vi "StackerStateMachine.vi"(0 "HMI to Control":T7, 1 "Arm Arrived":bool, 2 "StackClampState":T1, 5 "SensorInputData":T6, 7 "Intake Wheel State":T3, 9 "Tusk State":T4, 11 "error in":errorcluster) -> (4 "HMI to Control  Out":T7={"RightDriveValue"=0.0, "LeftDriveValue"=0.0, "Arm Manual "=0.0, "Stacker Manual "=0.0, "Claw Manual "=0.0, "ClawSlightOpenNumber"=0, "Intake Value "=0.0, "Arm States"=enum."4 Tote", "Claw States"=enum."Claw Manual ", "Intake Man. or Sense"=enum."Sensing", "Stacker in Manual?"=FALSE, "Drop Stack? "=FALSE, "Tusk Up Request"=FALSE, "Tusk Down Request"=FALSE, "Inver. Wheels  In Request"=FALSE, "Inverse. Wheels Out Request "=FALSE, "Get Out of Manual Control"=FALSE, "Exit Score State"=FALSE, "DriveStraight Help?"=FALSE, "Stacker Shut Off No."=0, "Stacker Need Off?"=FALSE, "Collecting?"=FALSE, "Go to Hover"=FALSE, "Stack Clamp Lock "=FALSE, "Stack Clamp Unlock "=FALSE, "Claw Intake Value "=0.0, "Stack Clamp Lock No. "=0}, 6 "SensorInputData out":T6, 8 "# of Totes Out":i32, 10 "Stacker State to Index":T5=enum."Hold", 12 "Tusk State to Actuate":T4, 13 "StackClampState to Actuate":T1, 14 "Intake Wheel State to Actuate":T3, 15 "error out":errorcluster)   [LabVIEW 2014]
uses:
  Typedefs/StackerStates.ctl
  Typedefs/HMI_to_Control.ctl
  Typedefs/Arm States.ctl
  Typedefs/ClawStates.ctl
  Typedefs/IntakeWheelSenseOrManual.ctl
  Typedefs/SensorInputData.ctl
  Typedefs/TuskStates.ctl
  Typedefs/IntakeWheelStates.ctl
  Typedefs/StackClampStates.ctl
  Typedefs/ClawStateMachine.ctl
  Gensubs/Bert_or_Ernie.vi
panel:
  in  "Ernie Needed Ranges":T2={"5 on ground upper range"=196.0, "5 on ground lower range"=182.0, "6 on ground upper range"=220.0, "6 on ground on lower range"=200.0, "Hold 4 Up Limit"=17.2, "Hold 4 Low Limit "=10.0, "Hold 5 Up Limit"=15.7, "Hold 5 Low Limit"=10.0, "Get Tote Upper Ok Range "=0.6, "Get Tote Lower Ok Range"=-2.0, "Drop Stack Upper Ok Range"=0.3, "Drop Stack Lower Ok Range"=-0.5, "6 Tote Cal Upper Range"=90.0, "6 Tote Cal Lower Range"=85.0, "5 Tote Cal Upper Range "=90.0, "5 Tote Cal Lower Range "=76.0, "Stacker on Ground Bottom #"=1.5, "Hold 4 on Ground Upper Range  "=172.0, "4 on ground U.R"=174.0, "4 on ground L.R"=165.0} {"4 on ground L.R" format="%#_13g"; "4 on ground U.R" format="%#_13g"; "6 Tote Cal Upper Range" format="%#_13g"}
  in  "Bert Needed Ranges":T2={"5 on ground upper range"=193.0, "5 on ground lower range"=176.0, "6 on ground upper range"=212.0, "6 on ground on lower range"=204.0, "Hold 4 Up Limit"=21.0, "Hold 4 Low Limit "=10.0, "Hold 5 Up Limit"=18.5, "Hold 5 Low Limit"=10.5, "Get Tote Upper Ok Range "=0.7, "Get Tote Lower Ok Range"=-2.0, "Drop Stack Upper Ok Range"=0.5, "Drop Stack Lower Ok Range"=-0.5, "6 Tote Cal Upper Range"=90.0, "6 Tote Cal Lower Range"=85.0, "5 Tote Cal Upper Range "=90.0, "5 Tote Cal Lower Range "=54.0, "Stacker on Ground Bottom #"=1.5, "Hold 4 on Ground Upper Range  "=172.0, "4 on ground U.R"=174.0, "4 on ground L.R"=157.0} {"4 on ground L.R" format="%#_13g"; "4 on ground U.R" format="%#_13g"; "6 Tote Cal Upper Range" format="%#_13g"}
  out "Stacker State Out":T5=enum."Hold"
  out "Stacker State In":T5
  # "When to \nadvance\nto \nother ranges\n\nHas to match\nsetpoints\nin stacker\nsub vi"
  # "4 Bar checks\nmust be \nin line with\ncals\nin 4 bar\nsub vi"
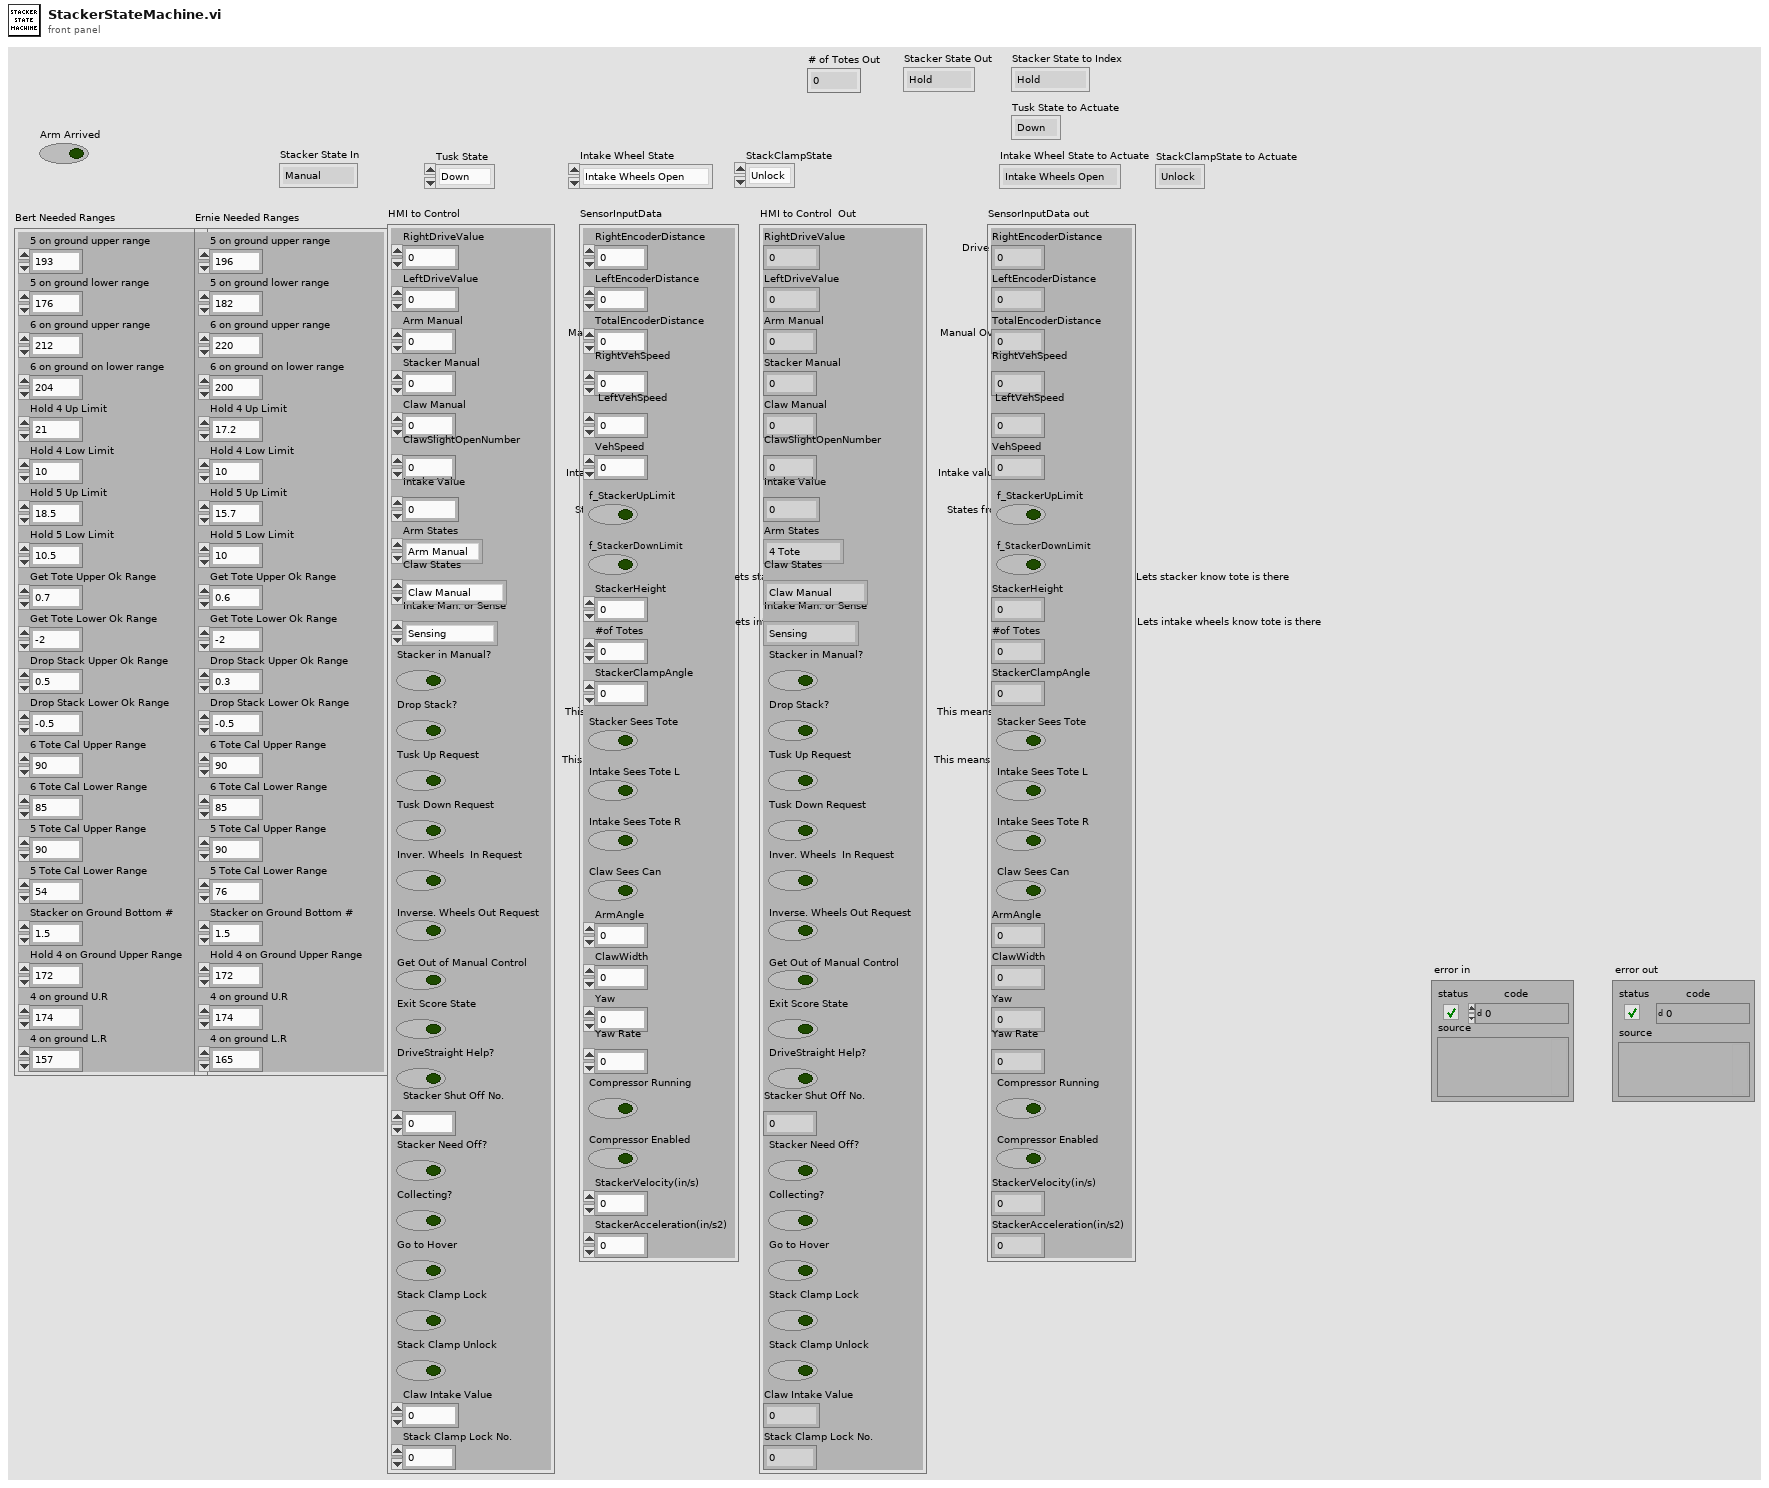
[diagram p1: front panel]
types:
  T1 = typedef "StackClampStates.ctl" = enum16{"Unlock", "Lock"}
  T2 = cluster{"5 on ground upper range":dbl, "5 on ground lower range":dbl, "6 on ground upper range":dbl, "6 on ground on lower range":dbl, "Hold 4 Up Limit":dbl, "Hold 4 Low Limit ":dbl, "Hold 5 Up Limit":dbl, "Hold 5 Low Limit":dbl, "Get Tote Upper Ok Range ":dbl, "Get Tote Lower Ok Range":dbl, "Drop Stack Upper Ok Range":dbl, "Drop Stack Lower Ok Range":dbl, "6 Tote Cal Upper Range":dbl, "6 Tote Cal Lower Range":dbl, "5 Tote Cal Upper Range ":dbl, "5 Tote Cal Lower Range ":dbl, "Stacker on Ground Bottom #":dbl, "Hold 4 on Ground Upper Range  ":dbl, "4 on ground U.R":dbl, "4 on ground L.R":dbl}
  T3 = typedef "IntakeWheelStates.ctl" = enum16{"Intake Wheels Open", "Intake Wheels Closed", "Decide off of Input", "Delay before Close", "Operator Request"}
  T4 = typedef "TuskStates.ctl" = enum16{"Down", "Up"}
  T5 = typedef "StackerStates.ctl" = enum16{"Manual ", "Hold", "Hold5", "Hold6", "GetTote", "DropStack", "Hover", "Hover5", "Wait for Up", "DecideHold", "DownTimerPeriod", "Prep Intake for Drop", "Check Arm before 5", "Make Arm ready for 5", "Check Arm before 6", "Make Arm ready for 6", "Delay for 5", "Delay for 6"}
  T6 = typedef "SensorInputData.ctl" = cluster{"RightEncoderDistance":dbl, "LeftEncoderDistance":dbl, "TotalEncoderDistance":dbl, "RightVehSpeed":dbl, "LeftVehSpeed":dbl, "VehSpeed":dbl, "f_StackerUpLimit":bool, "f_StackerDownLimit":bool, "StackerHeight":dbl, "#of Totes":u8, "StackerClampAngle":dbl, "Stacker Sees Tote":bool, "Intake Sees Tote L":bool, "Intake Sees Tote R":bool, "Claw Sees Can":bool, "ArmAngle":dbl, "ClawWidth":dbl, "Yaw":dbl, "Yaw Rate":dbl, "Compressor Running":bool, "Compressor Enabled":bool, "StackerVelocity(in/s)":dbl, "StackerAcceleration(in/s2)":dbl}
  T7 = typedef "HMI_to_Control.ctl" = cluster{"RightDriveValue":dbl, "LeftDriveValue":dbl, "Arm Manual ":dbl, "Stacker Manual ":dbl, "Claw Manual ":dbl, "ClawSlightOpenNumber":i8, "Intake Value ":sgl, "Arm States":T8, "Claw States":T9, "Intake Man. or Sense":T10, "Stacker in Manual?":bool, "Drop Stack? ":bool, "Tusk Up Request":bool, "Tusk Down Request":bool, "Inver. Wheels  In Request":bool, "Inverse. Wheels Out Request ":bool, "Get Out of Manual Control":bool, "Exit Score State":bool, "DriveStraight Help?":bool, "Stacker Shut Off No.":i8, "Stacker Need Off?":bool, "Collecting?":bool, "Go to Hover":bool, "Stack Clamp Lock ":bool, "Stack Clamp Unlock ":bool, "Claw Intake Value ":sgl, "Stack Clamp Lock No. ":i8}
  T8 = typedef "Arm States.ctl" = enum16{"Arm Manual ", "Ground", "Step", "1 Tote", "2 Tote", "3 Tote", "4 Tote", "5 Tote", "6 Tote", "Flip Can Arm", "Grab Can in auto", "Nudge"}
  T9 = typedef "ClawStates.ctl" = enum16{"Claw Manual ", "Claw Open", "Claw Closed", "Claw Slight Open", "Flip Can"}
  T10 = typedef "IntakeWheelSenseOrManual.ctl" = enum16{"Sensing", "Manual "}
  T11 = typedef "ClawStateMachine.ctl" = enum16{"Claw User Control", "Claw State Closed", "Claw State Slight Open"}
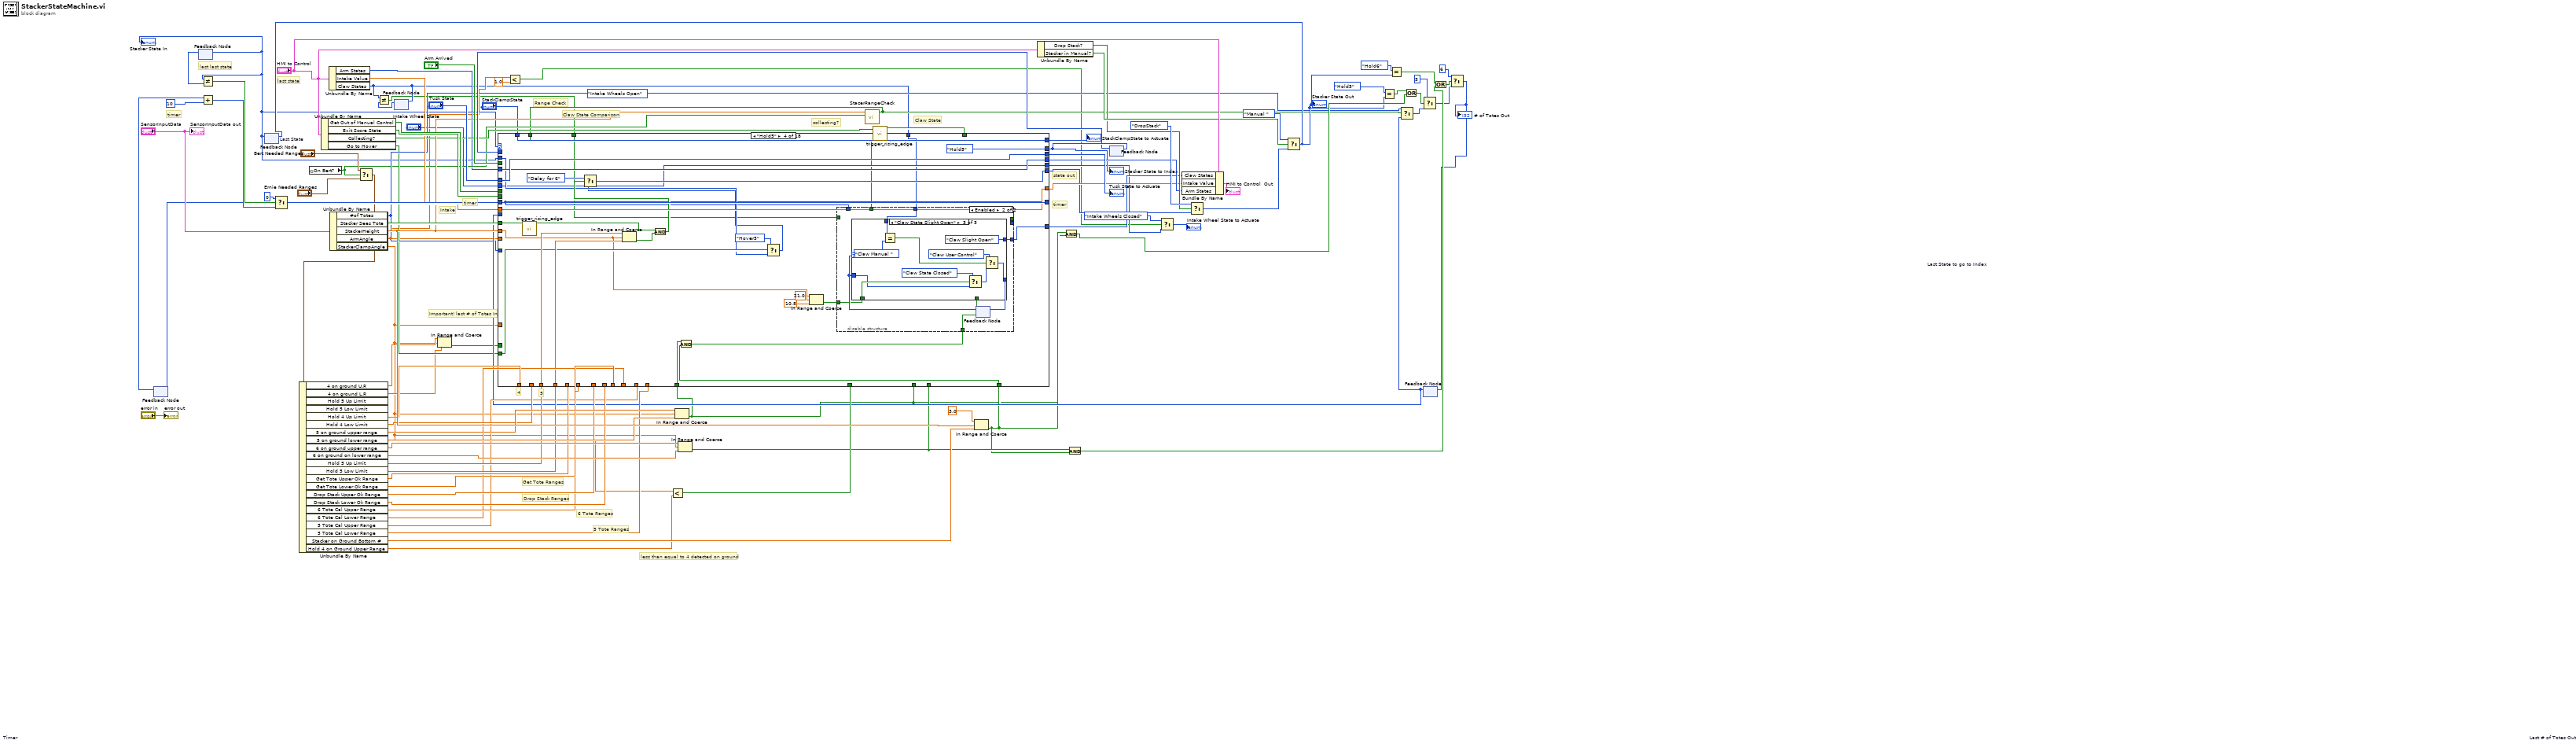
[diagram p0: block diagram]
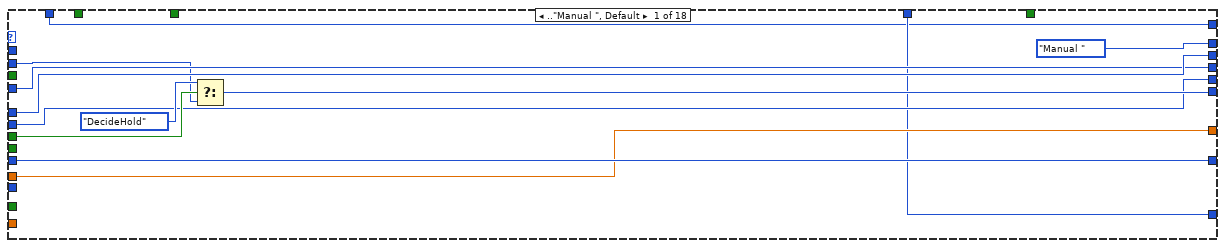
[diagram p2: hidden frame]
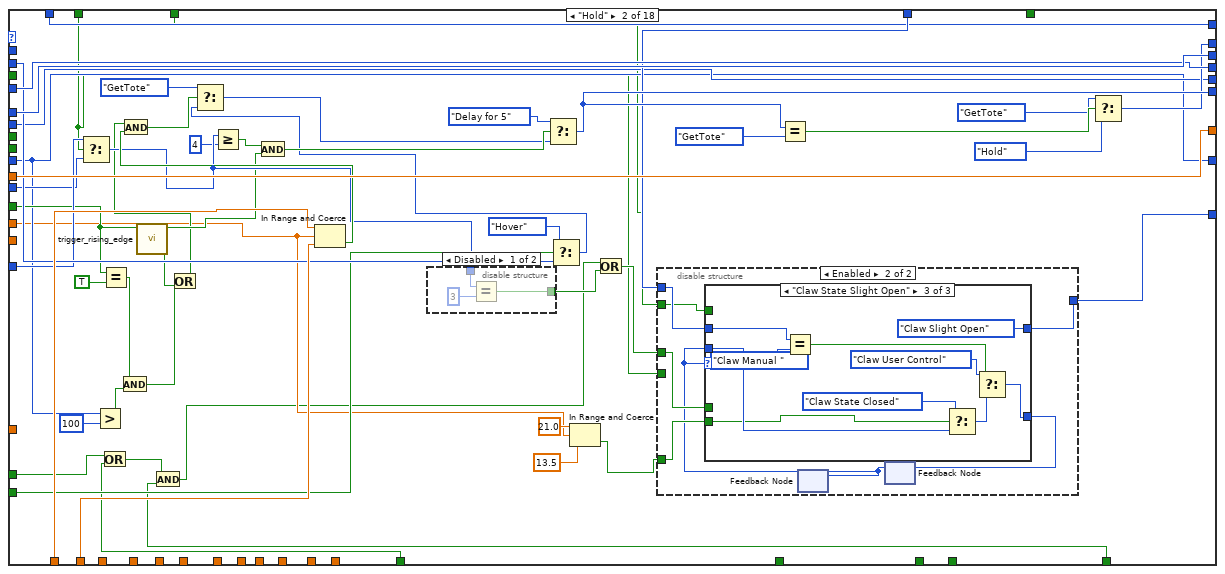
[diagram p3: hidden frame]
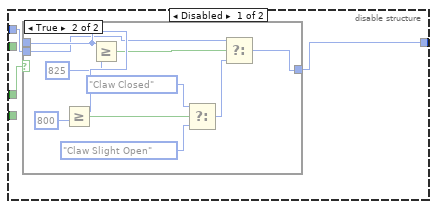
[diagram p4: hidden frame]
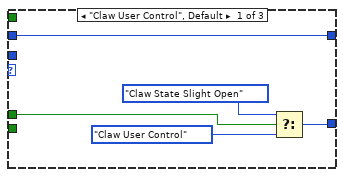
[diagram p6: hidden frame]
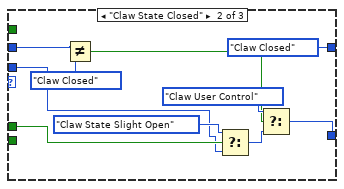
[diagram p7: hidden frame]
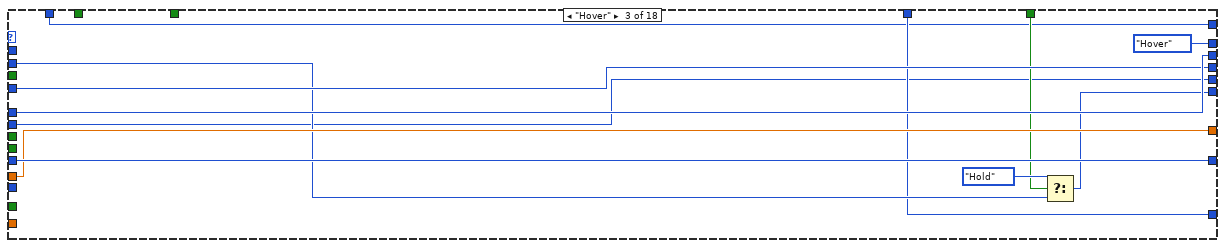
[diagram p9: hidden frame]
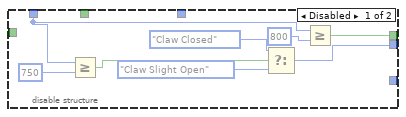
[diagram p10: hidden frame]
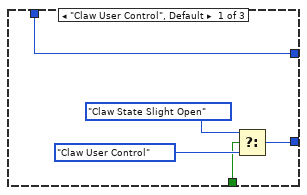
[diagram p11: hidden frame]
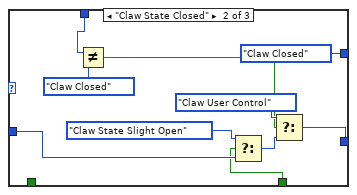
[diagram p12: hidden frame]
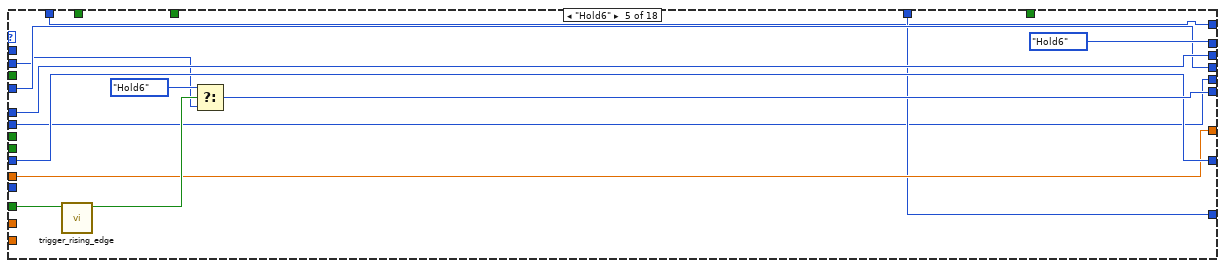
[diagram p13: hidden frame]
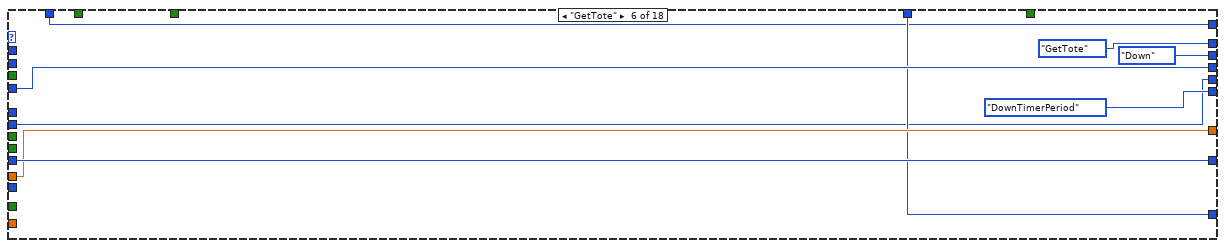
[diagram p14: hidden frame]
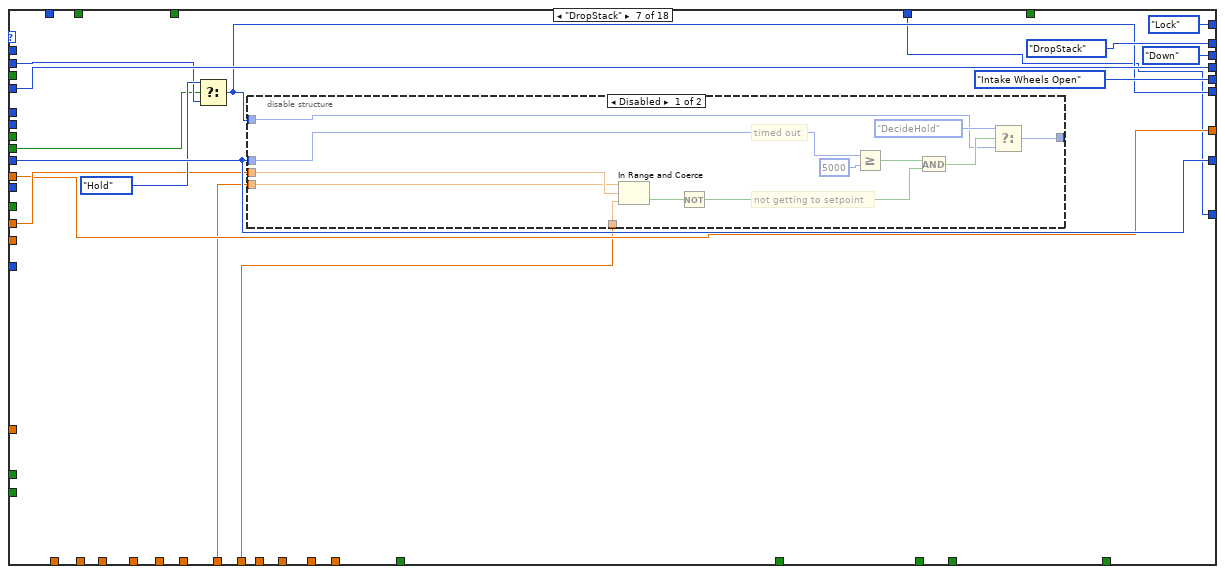
[diagram p15: hidden frame]
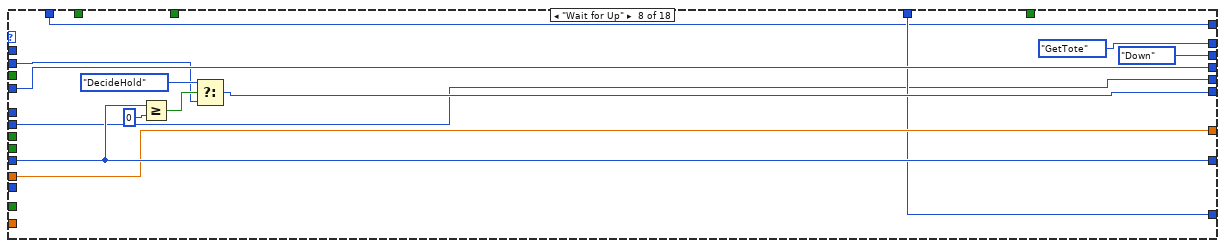
[diagram p17: hidden frame]
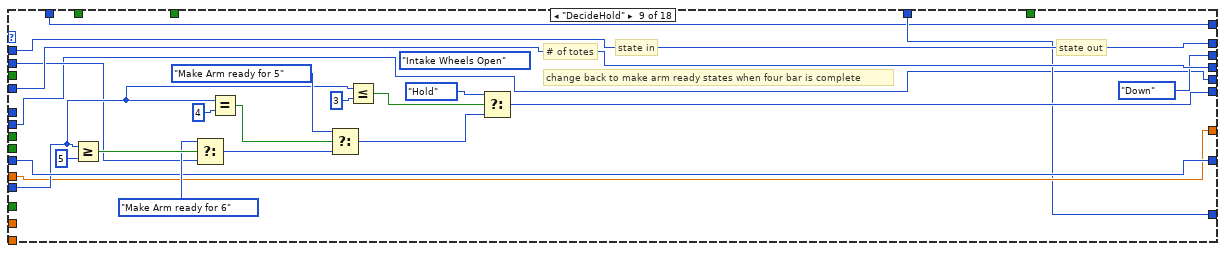
[diagram p18: hidden frame]
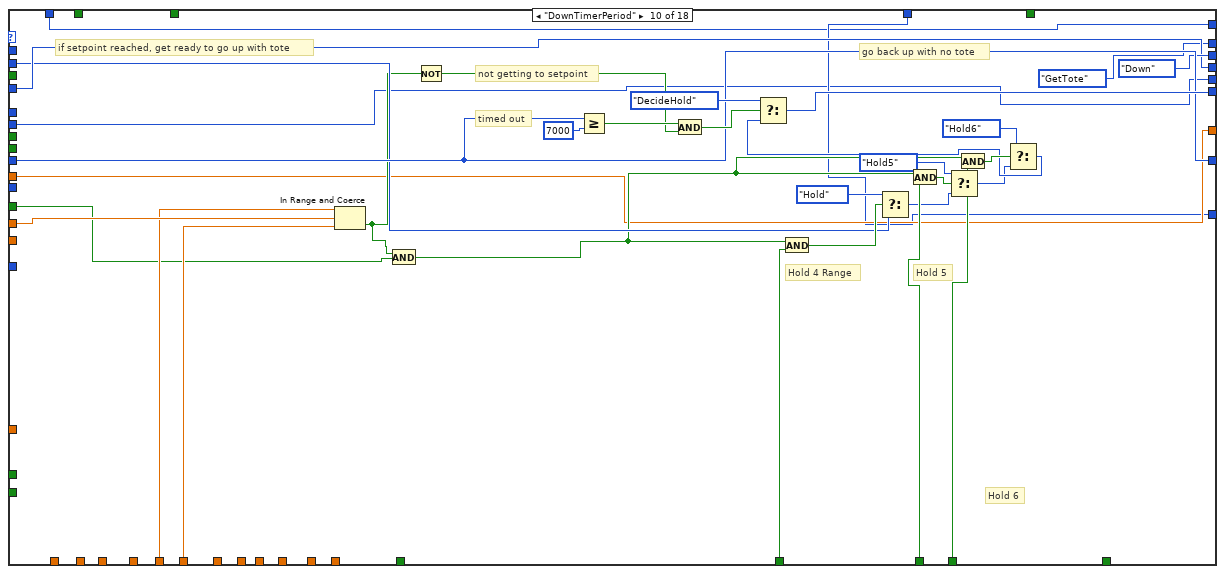
[diagram p19: hidden frame]
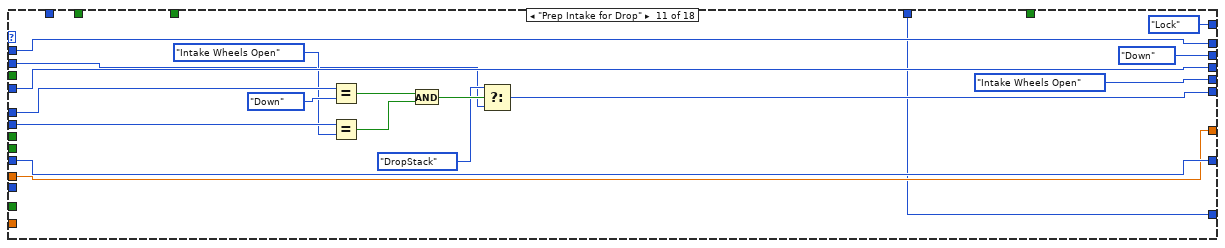
[diagram p20: hidden frame]
diagram:
  (unwired) IntakeWheelStates."Intake Wheels Open" ("y")
  # "Claw State Comparison"
  # "Range Check"
  # "Claw State"
  # "collecting?"
  # "less than equal to 4 detected on ground"
  # "5 Tote Ranges"
  # "6 Tote Ranges"
  # "Drop Stack Ranges"
  # "Get Tote Ranges"
  # "5"
  # "4"
  # "timer"
  # "state out"
  # "Important! last # of Totes In"
  # "Intake"
  # "timer"
  # "last state"
  # "last last state"
  # "timer"
  n1 = feedback #1 "Timer"() -> (w75:u32)  [unwired: 1 in]
  n2 = feedback #2() -> (w73:T5)  [unwired: 1 in]
  n3 = Add(x=w75, y=u32 10) -> (x+y=w91:u32)
  n4 = feedback #3 "Last State"() -> (w19:T5)  [unwired: 1 in]
  "Stacker State In" <- w19
  n5 = feedback-in #2(w19) -> ()
  n6 = Not Equal?(x=w19, y=w73) -> (x != y?=w90:bool)
  n7 = Select(t=u32 0, s=w90, f=w91) -> (s? t:f=w72:u32)
  n8 = global read "Bert_or_Ernie.vi" "On Bert?"() -> (w25:bool)
  n9 = Unbundle By Name("HMI to Control") -> ("Get Out of Manual Control"=w79:bool, "Exit Score State"=w78:bool, "Collecting?"=w29:bool, "Go to Hover"=w26:bool)
  n10 = Unbundle By Name("HMI to Control") -> ("Arm States"=w16:T8, "Intake Value"=w69:sgl, "Claw States"=w9:T9)
  n11 = Unbundle By Name("SensorInputData") -> ("#of Totes"=w27:u8, "Stacker Sees Tote"=w71:bool, "StackerHeight"=w67:dbl, "ArmAngle"=w12:dbl, "StackerClampAngle"=w2:dbl)
  n12 = Select(t="Bert Needed Ranges", s=w25, f="Ernie Needed Ranges") -> (s? t:f=w48:T2)
  n13 = Unbundle By Name(w48) -> ("4 on ground U.R"=w4:dbl, "4 on ground L.R"=w3:dbl, "Hold 4 Up Limit"=w61:dbl, "Hold 4 Low Limit"=w60:dbl, "5 on ground upper range"=w66:dbl, "5 on ground lower range"=w64:dbl, "6 on ground upper range"=w63:dbl, "6 on ground on lower range"=w62:dbl, "Hold 5 Up Limit"=w59:dbl, "Hold 5 Low Limit"=w58:dbl, "Get Tote Upper Ok Range"=w57:dbl, "Get Tote Lower Ok Range"=w56:dbl, "Drop Stack Upper Ok Range"=w55:dbl, "Drop Stack Lower Ok Range"=w54:dbl, "6 Tote Cal Upper Range"=w53:dbl, "6 Tote Cal Lower Range"=w52:dbl, "5 Tote Cal Upper Range"=w51:dbl, "5 Tote Cal Lower Range"=w50:dbl, "Stacker on Ground Bottom #"=w33:dbl, "Hold 4 on Ground Upper Range"=w32:dbl)  [unwired: 2 out]
  n14 = feedback-in #4(w9) -> ()
  n15 = feedback #4() -> (w8:T9)  [unwired: 1 in]
  n16 = Not Equal?(x=w9, y=w8) -> (x != y?=w7:bool)
  n17 = In Range and Coerce(upper limit=w4, x=w2, lower limit=w3) -> (In Range?=w6:bool)  [unwired: 1 out]
  n18 = Less?(x=w12, y=1.0) -> (x < y?=w10:bool)
  n19 = Less?(x=w2, y=w32) -> (x < y?=w31:bool)
  n20 = In Range and Coerce(upper limit=w66, x=w2, lower limit=w64) -> (In Range?=w1:bool)  [unwired: 1 out]
  n21 = In Range and Coerce(upper limit=w63, x=w2, lower limit=w62) -> (In Range?=w24:bool)  [unwired: 1 out]
  n22 = call "StacerRangeCheck.vi"("On Bert?"=w25, "Stacker"=w67) -> ("In ok range to count?"=w23:bool)  [unwired: 9 in]
  n23 = call "trigger_rising_edge.vi"("input"=w29) -> ("rising"=w21:bool)  [unwired: 10 in]
  n24 = In Range and Coerce(upper limit=3.0, x=w67, lower limit=w33) -> (In Range?=w5:bool)  [unwired: 1 out]
  n25 = Unbundle By Name("HMI to Control") -> ("Drop Stack?"=w84:bool, "Stacker in Manual?"=w88:bool)
  n26 = And(x=w5, y=w1) -> (x .and. y?=w45:bool)
  n27 = And(x=w24, y=w5) -> (x .and. y?=w36:bool)
  n28 = feedback #5 "Last State to go to Index"() -> (w74:T5)  [unwired: 1 in]
  n29 = feedback #6 "Last # of Totes Out"() -> (w28:i32)  [unwired: 1 in]
  n30 = case shown="\"Hold5\"" w19 {
    tunnel: [w105 w149 w213 w250 w302 StackerStates."DownTimerPeriod" ("Enum") w321 w349 w364 w403 w414 w431 w450 w472 w486 w512 w530 w554] -> w30
    tunnel: w71 -> [_ w129 _ w249 w299 _ _ _ _ w389 _ _ _ _ _ _ _ _]
    tunnel: w72 -> [w104 w126 w221 w235 w301 w312 w324 w348 w363 w401 w412 w430 w455 w470 w496 w511 w531 w545]
    tunnel: [w104 w126 w221 w235 w301 w312 w324 w348 w363 w401 w412 w430 w455 w470 w496 w511 w531 w545] -> w77
    tunnel: [StackerStates."Manual " ("State In 2") w145 StackerStates."Hover" ("t") StackerStates."Hold5" ("Enum") StackerStates."Hold6" ("Enum") StackerStates."GetTote" ("State In 2") StackerStates."DropStack" ("State In 2") StackerStates."GetTote" ("State In 2") w362 StackerStates."GetTote" ("State In 2") w413 StackerStates."GetTote" ("State In 2") w445 StackerStates."GetTote" ("State In 2") w481 w519 w527 StackerStates."Hover" ("t")] -> w76
    tunnel: "Tusk State" -> [w103 w159 w219 w251 w300 _ _ _ _ _ w422 _ _ _ _ w518 w526 w551]
    tunnel: "Intake Wheel State" -> [w102 w131 w210 w233 w291 w304 _ w340 w353 w375 w420 _ _ _ _ w516 w524 w538]
    tunnel: [w103 w159 w219 w251 w300 TuskStates."Down" ("Tusk State") TuskStates."Down" ("Tusk State") TuskStates."Down" ("Tusk State") TuskStates."Down" ("Tusk State") TuskStates."Down" ("Tusk State") TuskStates."Down" ("Tusk State") TuskStates."Down" ("Tusk State") TuskStates."Down" ("Tusk State") TuskStates."Down" ("Tusk State") TuskStates."Down" ("Tusk State") w518 w526 w551] -> w82
    tunnel: [w102 w131 w210 w233 w291 w304 IntakeWheelStates."Intake Wheels Open" ("Intake Wheel States") w340 w353 w375 IntakeWheelStates."Intake Wheels Open" ("Intake Wheel States") IntakeWheelStates."Intake Wheels Closed" ("Intake Wheel States") IntakeWheelStates."Intake Wheels Closed" ("Intake Wheel States") IntakeWheelStates."Intake Wheels Closed" ("Intake Wheel States") IntakeWheelStates."Intake Wheels Closed" ("Intake Wheel States") w516 w524 w538] -> w14
    tunnel: w74 -> [_ _ _ _ _ _ _ _ w362 _ w413 _ w446 _ w482 w519 w527 _]
    tunnel: w16 -> [w101 w158 w218 w246 w295 w308 w326 w345 w361 w399 w425 w433 w460 w473 w493 w517 w525 w552]
    tunnel: [w101 w158 w218 w246 w295 w308 w326 w345 w361 w399 w425 w429 w458 w469 w497 w517 w525 w552] -> w81
    tunnel: "Arm Arrived" -> [_ _ _ _ _ _ _ _ _ _ _ _ _ _ _ _ _ _]
    tunnel: w79 -> [w107 _ _ _ _ _ _ _ _ _ _ _ _ _ _ _ _ _]
    tunnel: w67 -> [_ w118 _ w224 _ _ w322 _ _ w398 _ _ _ _ _ w507 w528 _]
    tunnel: w78 -> [_ _ _ _ _ _ w314 _ _ _ _ _ _ _ _ _ _ _]
    tunnel: w28 -> [_ w136 _ _ _ _ _ _ w359 _ _ _ _ _ _ _ _ _]
    tunnel: [w100 w157 w217 w248 w297 w307 w320 w343 w356 w381 w411 w428 w454 w466 w492 w515 w529 w553] -> w70
    tunnel: w69 -> [w100 w157 w217 w248 w297 w307 w320 w343 w356 w381 w411 w428 w454 w466 w492 w515 w529 w553]
    tunnel: w12 -> [_ _ _ _ _ _ _ _ _ _ _ _ w453 _ w491 _ _ _]
    tunnel: w19 -> [w99 w142 w215 w237 w294 _ w319 w344 w357 w392 w410 _ w451 _ w489 w506 w532 w555]
    tunnel: w61 -> [_ w151 _ _ _ _ _ _ _ _ _ _ _ _ _ w505 _ _]
    tunnel: w60 -> [_ w150 _ _ _ _ _ _ _ _ _ _ _ _ _ w504 _ _]
    tunnel: w59 -> [_ _ _ w244 _ _ _ _ _ _ _ _ _ _ _ _ w523 _]
    tunnel: w58 -> [_ _ _ w243 _ _ _ _ _ _ _ _ _ _ _ _ w522 _]
    tunnel: w57 -> [_ _ _ _ _ _ _ _ _ w396 _ _ _ _ _ _ _ _]
    tunnel: w56 -> [_ _ _ _ _ _ _ _ _ w395 _ _ _ _ _ _ _ _]
    tunnel: w55 -> [_ _ _ _ _ _ w318 _ _ _ _ _ _ _ _ _ _ _]
    tunnel: w54 -> [_ _ _ _ _ _ w317 _ _ _ _ _ _ _ _ _ _ _]
    tunnel: w53 -> [_ _ _ _ _ _ _ _ _ _ _ _ w444 _ w488 _ _ _]
    tunnel: w52 -> [_ _ _ _ _ _ _ _ _ _ _ _ w443 _ w487 _ _ _]
    tunnel: w51 -> [_ _ _ _ _ _ _ _ _ _ _ _ _ _ _ _ _ _]
    tunnel: w50 -> [_ _ _ _ _ _ _ _ _ _ _ _ _ _ _ _ _ _]
    tunnel: w31 -> [_ _ _ _ _ _ _ _ _ w394 _ _ _ _ _ _ _ _]
    tunnel: w1 -> [_ _ _ _ _ _ _ _ _ w383 _ _ _ _ _ _ _ _]
    tunnel: w24 -> [_ _ _ _ _ _ _ _ _ w384 _ _ _ _ _ _ _ _]
    tunnel: w21 -> [_ _ w214 _ _ _ _ _ _ _ _ _ _ _ _ _ _ w556]
    tunnel: w27 -> [_ w137 _ _ _ _ _ _ _ _ _ _ _ _ _ _ _ _]
    tunnel: w26 -> [_ w140 _ w238 _ _ _ _ _ _ _ _ _ _ _ _ _ _]
    tunnel: [w98 w138 w212 w222 w293 w306 w315 w342 w355 w377 w409 w427 w442 w465 w480 w503 w521 w540] -> w20
    tunnel: w9 -> [w98 w139 w212 w230 w293 w306 w315 w342 w355 w377 w409 w427 w442 w465 w480 w503 w521 w541]
    tunnel: w23 -> [_ w121 _ w232 _ _ _ _ _ _ _ _ _ _ _ _ _ _]
    tunnel: "StackClampState" -> [w97 w132 w211 w234 w292 w305 _ w341 w354 w376 _ w426 w441 w464 w479 w502 w520 w539]
    tunnel: [w97 w132 w211 w234 w292 w305 StackClampStates."Lock" ("StackClampState") w341 w354 w376 StackClampStates."Lock" ("StackClampState") w426 w441 w464 w479 w502 w520 w539] -> w17
    tunnel: w7 -> [_ w122 _ w231 _ _ _ _ _ _ _ _ _ _ _ _ _ _]
    tunnel: w6 -> [_ w112 _ _ _ _ _ _ _ _ _ _ _ _ _ _ _ _]
    tunnel: w5 -> [_ w117 _ w229 _ _ _ _ _ _ _ _ _ _ _ _ _ _]
    tunnel: w2 -> [_ _ _ _ _ _ _ _ _ _ _ _ _ _ _ _ _ _]
    tunnel: w1 -> [_ w110 _ w223 _ _ _ _ _ _ _ _ _ _ _ _ _ _]
    frame .."Manual ", Default {
      n31 = Select(t=StackerStates."DecideHold" ("State In 2"), s=w107, f=w99) -> (s? t:f=w105:T5)
    }
    frame "Hold" {
      n32 = Select(t=w137, s=w121, f=w136) -> (s? t:f=w135:i32)
      n33 = Greater?(x=w126, y=u32 100) -> (0:w113:bool)
      n34 = Or(x=w112, y=w110) -> (x .or. y?=w111:bool)
      n35 = Equal?(x=w129, y=TRUE) -> (x = y?=w127:bool)
      n36 = And(x=w127, y=w113) -> (x .and. y?=w124:bool)
      n37 = call "trigger_rising_edge.vi"("input"=w129) -> ("rising"=w130:bool)  [unwired: 10 in]
      n38 = And(x=w111, y=w117) -> (x .and. y?=w114:bool)
      n39 = Or(x=w124, y=w130) -> (x .or. y?=w123:bool)
      n40 = Greater Or Equal?(x=w135, y=u8 4) -> (x >= y?=w116:bool)
      n41 = And(x=w116, y=w130) -> (x .and. y?=w156:bool)
      n42 = In Range and Coerce(upper limit=w151, x=w118, lower limit=w150) -> (In Range?=w154:bool)  [unwired: 1 out]
      n43 = And(x=w123, y=w154) -> (x .and. y?=w153:bool)
      n44 = disable-structure shown="Disabled" {
        disable-tunnel: w135 -> [w209 _]
        disable-tunnel: [w208 _] -> w134
        frame Disabled {
          n45 = Equal?(x=w209, y=3) -> (x = y?=w208:bool)
        }
        frame Enabled {
        }
      }
      n46 = Select(t=StackerStates."Hover" ("y"), s=w140, f=w142) -> (s? t:f=w141:T5)
      n47 = Select(t=StackerStates."GetTote" ("State In 2"), s=w153, f=w141) -> (s? t:f=w155:T5)
      n48 = Select(t=StackerStates."Delay for 5" ("State In 2"), s=w156, f=w155) -> (s? t:f=w149:T5)
      n49 = In Range and Coerce(upper limit=21.0, x=w118, lower limit=13.5) -> (In Range?=w109:bool)  [unwired: 1 out]
      n50 = Or(x=w114, y=w134) -> (x .or. y?=w133:bool)
      n51 = disable-structure shown="Enabled" {
        disable-tunnel: w139 -> [w163 w181]
        disable-tunnel: [w162 w180] -> w138
        disable-tunnel: w133 -> [w161 w179]
        disable-tunnel: w122 -> [_ w176]
        disable-tunnel: w121 -> [_ _]
        disable-tunnel: w109 -> [_ w177]
        frame Disabled {
          n52 = case shown="True" w161 {
            tunnel: w163 -> [w164 w166]
            tunnel: _ -> [_ w170]
            tunnel: [w164 w165] -> w162
            frame False {
            }
            frame True {
              n53 = Greater Or Equal?(x=w170, y=u32 800) -> (x >= y?=w171:bool)
              n54 = Greater Or Equal?(x=w170, y=u32 825) -> (x >= y?=w168:bool)
              n55 = Select(t=ClawStates."Claw Closed" ("Claw States"), s=w171, f=ClawStates."Claw Slight Open" ("Claw States")) -> (s? t:f=w167:T9)
              n56 = Select(t=w166, s=w168, f=w167) -> (s? t:f=w165:T9)
            }
          }
        }
        frame Enabled {
          n57 = feedback #7() -> ()  [unwired: 2 in]
          n58 = feedback #8() -> (w175:T11)  [unwired: 1 in]
          n59 = case shown="\"Claw State Slight Open\"" w175 {
            tunnel: w181 -> [w186 w189 w202]
            tunnel: [w186 ClawStates."Claw Closed" ("Claw States") ClawStates."Claw Slight Open" ("Claw States")] -> w180
            tunnel: w179 -> [w184 w192 _]
            tunnel: [w182 w190 w197] -> w178
            tunnel: w177 -> [_ _ w203]
            tunnel: w175 -> [_ w191 w205]
            tunnel: w176 -> [_ _ _]
            frame "Claw User Control", Default {
              n60 = Select(t=ClawStateMachine."Claw State Slight Open", s=w184, f=ClawStateMachine."Claw User Control") -> (s? t:f=w182:T11)
            }
            frame "Claw State Closed" {
              n61 = Not Equal?(x=w189, y=ClawStates."Claw Closed") -> (x != y?=w187:bool)
              n62 = Select(t=ClawStateMachine."Claw State Slight Open", s=w192, f=w191) -> (s? t:f=w193:T11)
              n63 = Select(t=ClawStateMachine."Claw User Control", s=w187, f=w193) -> (s? t:f=w190:T11)
            }
            frame "Claw State Slight Open" {
              n64 = Equal?(x=w202, y=ClawStates."Claw Manual ") -> (x = y?=w198:bool)
              n65 = Select(t=ClawStateMachine."Claw State Closed", s=w203, f=w205) -> (s? t:f=w200:T11)
              n66 = Select(t=ClawStateMachine."Claw User Control", s=w198, f=w200) -> (s? t:f=w197:T11)
            }
          }
          n67 = feedback-in #7(w175) -> ()
          n68 = feedback-in #8(w178) -> ()
        }
      }
      n69 = Equal?(x=w149, y=StackerStates."GetTote") -> (x = y?=w147:bool)
      n70 = Select(t=StackerStates."GetTote" ("y"), s=w147, f=StackerStates."Hold" ("State In 2")) -> (s? t:f=w145:T5)
    }
    frame "Hover" {
      n71 = Select(t=StackerStates."Hold", s=w214, f=w215) -> (s? t:f=w213:T5)
    }
    frame "Hold5" {
      n72 = call "trigger_rising_edge.vi"("input"=w249) -> ("rising"=w241:bool)  [unwired: 10 in]
      n73 = In Range and Coerce(upper limit=w244, x=w224, lower limit=w243) -> (In Range?=w242:bool)  [unwired: 1 out]
      n74 = And(x=w241, y=w242) -> (x .and. y?=w240:bool)
      n75 = And(x=w223, y=w229) -> (x .and. y?=w228:bool)
      n76 = Select(t=StackerStates."Hover5" ("y"), s=w238, f=w237) -> (s? t:f=w236:T5)
      n77 = Select(t=StackerStates."Delay for 6" ("Enum"), s=w240, f=w236) -> (s? t:f=w250:T5)
      n78 = In Range and Coerce(upper limit=21.0, x=w224, lower limit=10.8) -> (In Range?=w225:bool)  [unwired: 1 out]
      n79 = disable-structure shown="Enabled" {
        disable-tunnel: w235 -> [w255 _]
        disable-tunnel: [w253 _] -> _
        disable-tunnel: [w252 _] -> _
        disable-tunnel: w232 -> [_ _]
        disable-tunnel: w231 -> [_ _]
        disable-tunnel: w230 -> [_ w265]
        disable-tunnel: w228 -> [_ w264]
        disable-tunnel: w225 -> [_ w261]
        disable-tunnel: [_ w260] -> w222
        frame Disabled {
          n80 = Greater Or Equal?(x=w255, y=u32 750) -> (x >= y?=w258:bool)
          n81 = Select(t=ClawStates."Claw Closed" ("Claw States"), s=w258, f=ClawStates."Claw Slight Open") -> (s? t:f=w252:T9)
          n82 = Greater Or Equal?(x=w255, y=u32 800) -> (x >= y?=w253:bool)
        }
        frame Enabled {
          n83 = feedback #9() -> (w262:T11)  [unwired: 1 in]
          n84 = case shown="\"Claw State Slight Open\"" w262 {
            tunnel: [w266 ClawStates."Claw Closed" ("Claw States") ClawStates."Claw Slight Open" ("Claw States")] -> w260
            tunnel: [w268 w276 w281] -> w263
            tunnel: w265 -> [w266 w273 w286]
            tunnel: w264 -> [w267 w271 _]
            tunnel: w262 -> [_ w272 w287]
            tunnel: w261 -> [_ _ w288]
            frame "Claw User Control", Default {
              n85 = Select(t=ClawStateMachine."Claw State Slight Open", s=w267, f=ClawStateMachine."Claw User Control") -> (s? t:f=w268:T11)
            }
            frame "Claw State Closed" {
              n86 = Not Equal?(x=w273, y=ClawStates."Claw Closed") -> (x != y?=w274:bool)
              n87 = Select(t=ClawStateMachine."Claw State Slight Open", s=w271, f=w272) -> (s? t:f=w277:T11)
              n88 = Select(t=ClawStateMachine."Claw User Control", s=w274, f=w277) -> (s? t:f=w276:T11)
            }
            frame "Claw State Slight Open" {
              n89 = Equal?(x=w286, y=ClawStates."Claw Manual ") -> (x = y?=w283:bool)
              n90 = Select(t=ClawStateMachine."Claw State Closed", s=w288, f=w287) -> (s? t:f=w282:T11)
              n91 = Select(t=ClawStateMachine."Claw User Control", s=w283, f=w282) -> (s? t:f=w281:T11)
            }
          }
          n92 = feedback-in #9(w263) -> ()
        }
      }
    }
    frame "Hold6" {
      n93 = call "trigger_rising_edge.vi"("input"=w299) -> ("rising"=w298:bool)  [unwired: 10 in]
      n94 = Select(t=StackerStates."Hold6" ("State Out 2"), s=w298, f=w294) -> (s? t:f=w302:T5)
    }
    frame "GetTote" {
    }
    frame "DropStack" {
      n95 = Select(t=StackerStates."Hold" ("Enum"), s=w314, f=w319) -> (s? t:f=w321:T5)
      n96 = disable-structure shown="Disabled" {
        disable-tunnel: [w333 _] -> _
        disable-tunnel: w324 -> [w332 _]
        disable-tunnel: w321 -> [w331 _]
        disable-tunnel: w322 -> [w330 _]
        disable-tunnel: w318 -> [w329 _]
        disable-tunnel: w317 -> [w328 _]
        frame Disabled {
          # "not getting to setpoint"
          # "timed out"
          n97 = In Range and Coerce(upper limit=w329, x=w330, lower limit=w328) -> (In Range?=w335:bool)  [unwired: 1 out]
          n98 = Not(x=w335) -> (.not. x?=w337:bool)
          n99 = Greater Or Equal?(x=w332, y=u32 5000) -> (x >= y?=w339:bool)
          n100 = And(x=w339, y=w337) -> (x .and. y?=w338:bool)
          n101 = Select(t=StackerStates."DecideHold" ("Stacker State In 2"), s=w338, f=w331) -> (s? t:f=w333:T5)
        }
        frame Enabled {
        }
      }
    }
    frame "Wait for Up" {
      n102 = Greater Or Equal?(x=w348, y=u32 0) -> (x >= y?=w351:bool)
      n103 = Select(t=StackerStates."DecideHold" ("Stacker State In 2"), s=w351, f=w344) -> (s? t:f=w349:T5)
    }
    frame "DecideHold" {
      (unwired) IntakeWheelStates."Intake Wheels Open" ("Intake Wheel States")
      # "# of totes"
      # "change back to make arm ready states when four bar is complete"
      # "state out"
      # "state in"
      n104 = Greater Or Equal?(x=w359, y=i8 5) -> (x >= y?=w374:bool)
      n105 = Select(t=StackerStates."Make Arm ready for 6" ("State In 2"), s=w374, f=w357) -> (s? t:f=w372:T5)
      n106 = Equal?(x=w359, y=i8 4) -> (x = y?=w370:bool)
      n107 = Select(t=StackerStates."Make Arm ready for 5" ("State In 2"), s=w370, f=w372) -> (s? t:f=w367:T5)
      n108 = Less Or Equal?(x=w359, y=i8 3) -> (x <= y?=w365:bool)
      n109 = Select(t=StackerStates."Hold" ("State In 2"), s=w365, f=w367) -> (s? t:f=w364:T5)
    }
    frame "DownTimerPeriod" {
      # "Hold 5"
      # "Hold 6"
      # "Hold 4 Range"
      # "if setpoint reached, get ready to go up with tote"
      # "go back up with no tote"
      # "not getting to setpoint"
      # "timed out"
      n110 = In Range and Coerce(upper limit=w396, x=w398, lower limit=w395) -> (In Range?=w390:bool)  [unwired: 1 out]
      n111 = And(x=w390, y=w389) -> (x .and. y?=w385:bool)
      n112 = Not(x=w390) -> (.not. x?=w405:bool)
      n113 = Greater Or Equal?(x=w401, y=u32 7000) -> (x >= y?=w407:bool)
      n114 = And(x=w407, y=w405) -> (x .and. y?=w406:bool)
      n115 = And(x=w385, y=w394) -> (x .and. y?=w393:bool)
      n116 = Select(t=StackerStates."Hold", s=w393, f=w392) -> (s? t:f=w379:T5)
      n117 = And(x=w385, y=w383) -> (x .and. y?=w388:bool)
      n118 = Select(t=StackerStates."Hold5", s=w388, f=w379) -> (s? t:f=w380:T5)
      n119 = And(x=w385, y=w384) -> (x .and. y?=w386:bool)
      n120 = Select(t=StackerStates."Hold6", s=w386, f=w380) -> (s? t:f=w382:T5)
      n121 = Select(t=StackerStates."DecideHold" ("Stacker State In 2"), s=w406, f=w382) -> (s? t:f=w403:T5)
    }
    frame "Prep Intake for Drop" {
      n122 = Equal?(x=w422, y=TuskStates."Down") -> (x = y?=w418:bool)
      n123 = Equal?(x=w420, y=IntakeWheelStates."Intake Wheels Open") -> (x = y?=w417:bool)
      n124 = And(x=w418, y=w417) -> (x .and. y?=w416:bool)
      n125 = Select(t=StackerStates."DropStack" ("Enum"), s=w416, f=w410) -> (s? t:f=w414:T5)
    }
    frame "Check Arm before 5" {
      # "Arm State"
      # "Stacker State"
      # "timer"
      # "state to index"
      n126 = Equal?(x=w433, y=Arm_States."6 Tote") -> (x = y?=w436:bool)
      n127 = Select(t=w433, s=w436, f=Arm_States."6 Tote") -> (s? t:f=w429:T8)
      n128 = Select(t=StackerStates."Hold5" ("Enum"), s=w436, f=StackerStates."Make Arm ready for 5") -> (s? t:f=w431:T5)
    }
    frame "Make Arm ready for 5" {
      # "Stacker State"
      # "Arm State"
      # "timer"
      n129 = Equal?(x=w460, y=Arm_States."6 Tote") -> (x = y?=w461:bool)
      n130 = Select(t=w460, s=w461, f=Arm_States."6 Tote") -> (s? t:f=w458:T8)
      n131 = In Range and Coerce(upper limit=w444, x=w453, lower limit=w443) -> (In Range?=w452:bool)  [unwired: 1 out]
      n132 = Select(t=StackerStates."Hold5", s=w452, f=w451) -> (s? t:f=w450:T5)
      n133 = Equal?(x=StackerStates."Hold5", y=w450) -> (x = y?=w448:bool)
      n134 = Select(t=StackerStates."Hold5" ("x"), s=w448, f=w446) -> (s? t:f=w445:T5)
    }
    frame "Check Arm before 6" {
      n135 = Equal?(x=w473, y=Arm_States."6 Tote") -> (x = y?=w475:bool)
      n136 = Select(t=w473, s=w475, f=Arm_States."6 Tote") -> (s? t:f=w469:T8)
      n137 = Select(t=StackerStates."Hold6" ("Enum"), s=w475, f=StackerStates."Make Arm ready for 6") -> (s? t:f=w472:T5)
    }
    frame "Make Arm ready for 6" {
      n138 = In Range and Coerce(upper limit=w488, x=w491, lower limit=w487) -> (In Range?=w490:bool)  [unwired: 1 out]
      n139 = Equal?(x=w493, y=Arm_States."6 Tote") -> (x = y?=w499:bool)
      n140 = Select(t=w493, s=w499, f=Arm_States."6 Tote") -> (s? t:f=w497:T8)
      n141 = Select(t=StackerStates."Hold6", s=w490, f=w489) -> (s? t:f=w486:T5)
      n142 = Equal?(x=StackerStates."Hold6" ("t"), y=w486) -> (x = y?=w484:bool)
      n143 = Select(t=StackerStates."Hold6", s=w484, f=w482) -> (s? t:f=w481:T5)
    }
    frame "Delay for 5" {
      n144 = In Range and Coerce(upper limit=w505, x=w507, lower limit=w504) -> (In Range?=w508:bool)  [unwired: 1 out]
      n145 = Greater Or Equal?(x=w511, y=u32 0) -> (x >= y?=w510:bool)
      n146 = And(x=w510, y=w508) -> (x .and. y?=w509:bool)
      n147 = Select(t=StackerStates."GetTote" ("Enum"), s=w509, f=w506) -> (s? t:f=w512:T5)
    }
    frame "Delay for 6" {
      n148 = In Range and Coerce(upper limit=w523, x=w528, lower limit=w522) -> (In Range?=w537:bool)  [unwired: 1 out]
      n149 = Greater Or Equal?(x=w531, y=u32 0) -> (x >= y?=w535:bool)
      n150 = And(x=w535, y=w537) -> (x .and. y?=w536:bool)
      n151 = Select(t=StackerStates."GetTote" ("Enum"), s=w536, f=w532) -> (s? t:f=w530:T5)
    }
    frame "Hover5" {
      n152 = Greater Or Equal?(x=w545, y=u32 1000) -> (x >= y?=w543:bool)
      n153 = Greater Or Equal?(x=w545, y=u32 1050) -> (x >= y?=w542:bool)
      n154 = Select(t=ClawStates."Claw Closed" ("Claw States"), s=w543, f=ClawStates."Claw Slight Open" ("Claw States")) -> (s? t:f=w547:T9)
      n155 = Select(t=w541, s=w542, f=w547) -> (s? t:f=w540:T9)
      n156 = Select(t=StackerStates."Hold5", s=w556, f=w555) -> (s? t:f=w554:T5)
    }
  }
  "Stacker State to Index" <- w76
  "Tusk State to Actuate" <- w82
  "StackClampState to Actuate" <- w17
  n157 = feedback-in #1(w77) -> ()
  n158 = feedback-in #5(w76) -> ()
  n159 = Select(t=IntakeWheelStates."Intake Wheels Closed" ("Intake Wheel State"), s=w10, f=w14) -> (s? t:f=→"Intake Wheel State to Actuate":T3)
  n160 = Bundle By Name(cluster="HMI to Control", "Claw States"=w20, "Intake Value"=w70, "Arm States"=w81) -> (→"HMI to Control  Out":T7)
  n161 = Select(t=StackerStates."DropStack", s=w84, f=w30) -> (s? t:f=w87:T5)
  n162 = Select(t=StackerStates."Manual ", s=w88, f=w87) -> (s? t:f=w39:T5)
  "Stacker State Out" <- w39
  n163 = feedback-in #3(w39) -> ()
  n164 = Equal?(x=StackerStates."Hold5" ("y"), y=w39) -> (x = y?=w46:bool)
  n165 = Equal?(x=StackerStates."Hold6" ("y"), y=w39) -> (x = y?=w38:bool)
  n166 = Select(t=w27, s=w23, f=w28) -> (s? t:f=w42:i32)
  n167 = Or(x=w46, y=w45) -> (x .or. y?=w44:bool)
  n168 = Select(t=5, s=w44, f=w42) -> (s? t:f=w35:i32)
  n169 = Or(x=w38, y=w36) -> (x .or. y?=w37:bool)
  n170 = Select(t=6, s=w37, f=w35) -> (s? t:f=w34:i32)
  "# of Totes Out" <- w34
  n171 = feedback-in #6(w34) -> ()
  "SensorInputData out" <- "SensorInputData"
  "error out" <- "error in"
